vi "SkySparkCallForgetAcq.vi"(8 "error in (no error)":errorcluster, 11 "SkySparkDevice in":refnum<class "SkySparkDevice.lvclass">) -> (0 "error out":errorcluster, 2 "FGV_Cluster Output":T1, 3 "SkySparkDevice out":refnum<class "SkySparkDevice.lvclass">)   [LabVIEW 2020, in "SkySparkDevice.lvclass"]
uses:
  SkySparkDevice.lvclass
  FGV_TypeDef.ctl
  FGVFunctionTypeDef.ctl
  AcquireHardware2.vi
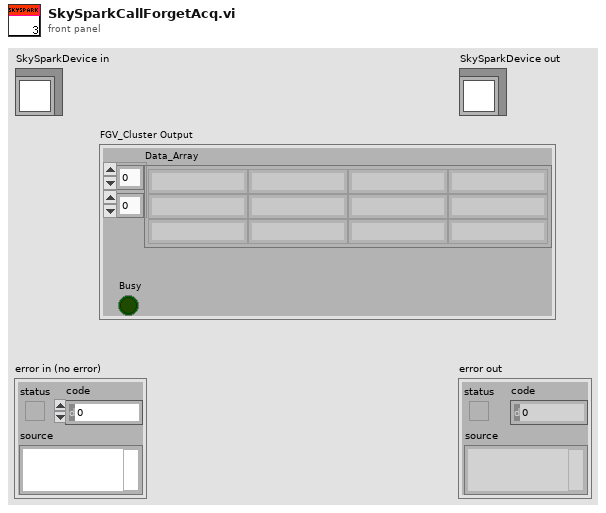
[diagram p1: front panel]
types:
  T1 = typedef "SkySparkDevice.lvclass/FGV_TypeDef.ctl" = cluster{"Data_Array":string[][], "Busy":bool}
  T2 = typedef "SkySparkDevice.lvclass/FGVFunctionTypeDef.ctl" = enum16{"Clear", "Write", "Read"}
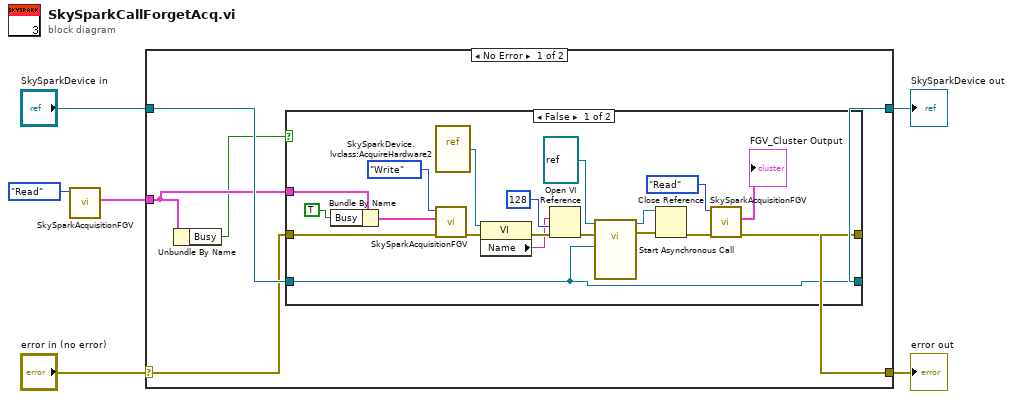
[diagram p0: block diagram]
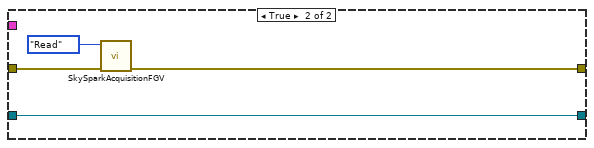
[diagram p2: hidden frame]
diagram:
  n1 = call "SkySparkAcquisitionFGV.vi"("Function"=FGVFunctionTypeDef."Read") -> ("FGV_Cluster Output"=w1:T1)  [unwired: 9 in, 1 out]
  n2 = case shown="No Error" "error in (no error)" {
    selector: "error in (no error)" -> [w10 w37]
    tunnel: [w9 w37] -> w5
    tunnel: [w11 w36] -> w3
    tunnel: "SkySparkDevice in" -> [w12 w36]
    tunnel: w1 -> [w8 _]
    frame No Error {
      n3 = Unbundle By Name(w8) -> ("Busy"=w7:bool)
      n4 = case shown="False" w7 {
        tunnel: w12 -> [w15 w32]
        tunnel: [w15 w32] -> w11
        tunnel: w10 -> [w23 w34]
        tunnel: [w20 w33] -> w9
        tunnel: w8 -> [w31 _]
        frame False {
          n5 = Bundle By Name(cluster=w31, "Busy"=TRUE) -> (w29:T1)
          n6 = vi-ref "SkySparkDevice.lvclass:AcquireHardware2.vi"() -> (w13:refnum<vi>)
          n7 = call "SkySparkAcquisitionFGV.vi"("error in (no error)"=w23, "FGV_Cluster Input"=w29, "Function"=FGVFunctionTypeDef."Write") -> ("error out"=w27:errorcluster)  [unwired: 7 in, 1 out]
          n8 = property class="VI"(reference=w13, error in=w27) -> (error out=w25:errorcluster, "Name"=w24:string)  [unwired: 1 out]
          n9 = Open VI Reference(vi path=w24, options=128, error in (no error)=w25) -> (error out=w19:errorcluster)  [unwired: 3 in, 1 out]
          n10 = call-by-ref "Start Asynchronous Call"(reference=refnum<vi> refnum, error in=w19, "SkySparkDevice in"=w15) -> (reference out=w17:refnum<vi>, error out=w18:errorcluster)  [unwired: 9 in, 2 out]
          n11 = Close Reference(reference=w17, error in (no error)=w18) -> (error out=w21:errorcluster)
          n12 = call "SkySparkAcquisitionFGV.vi"("error in (no error)"=w21, "Function"=FGVFunctionTypeDef."Read") -> ("error out"=w20:errorcluster, "FGV_Cluster Output"=→"FGV_Cluster Output":T1)  [unwired: 8 in]
        }
        frame True {
          n13 = call "SkySparkAcquisitionFGV.vi"("error in (no error)"=w34, "Function"=FGVFunctionTypeDef."Read") -> ("error out"=w33:errorcluster)  [unwired: 8 in, 1 out]
        }
      }
    }
    frame Error {
    }
  }
  "error out" <- w5
  "SkySparkDevice out" <- w3
